vi "Init Msg Input.vi"(6 "Teller":refnum<class "Teller.lvclass">, 9 "Error":errorcluster, 10 "Actor":refnum<class "Actor.lvclass">) -> (3 "Stopped Msg Input out":refnum<class "Stopped Msg Input.lvclass">)   [LabVIEW 2025, in "jettl.lvlib" / "Stopped jettl Msg.lvlib" / "Stopped Msg Input.lvlib" / "Stopped Msg Input.lvclass"]
uses:
  Stopped Msg Input.lvclass
  Actor/Actor.lvclass
  Teller/Teller.lvclass
  Stopped Msg Input.lvclass/Stopped Msg Input.ctl
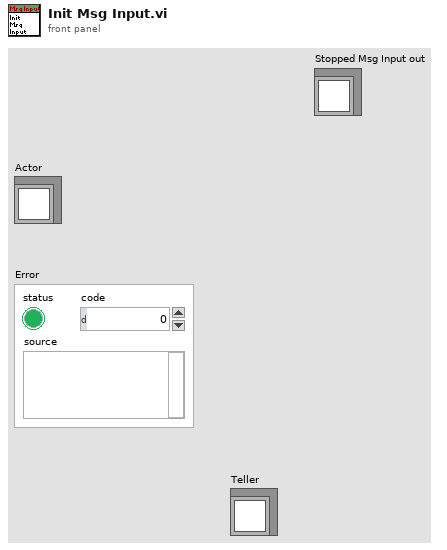
[diagram p1: front panel]
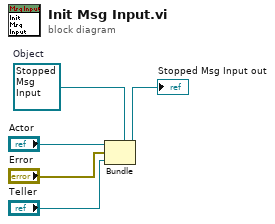
[diagram p0: block diagram]
diagram:
  w5 = refnum<class "Stopped Msg Input.lvclass"> refnum  # Object
  n1 = Bundle "Bundle"(cluster=w5, "Actor", "Error", "Teller") -> (→"Stopped Msg Input out":refnum<class "Stopped Msg Input.lvclass">)
